vi "Teleop_Calc_Distance.vi"(11 "Teleop Local Data in":T1) -> (3 "Teleop Local Data out":T1)   [LabVIEW 2016]
uses:
  Typedefs/typedef_cluster_Teleop Local Data.ctl
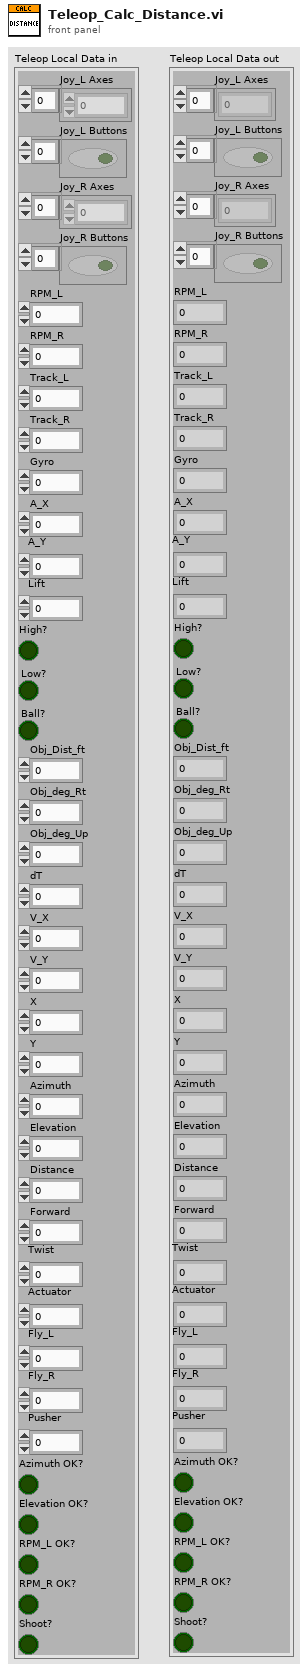
[diagram p1: front panel]
types:
  T1 = typedef "typedef_cluster_Teleop Local Data.ctl" = cluster{"Joy_L Axes":dbl[], "Joy_L Buttons":bool[], "Joy_R Axes":dbl[], "Joy_R Buttons":bool[], "RPM_L":dbl, "RPM_R":dbl, "Track_L":dbl, "Track_R":dbl, "Gyro":dbl, "A_X":dbl, "A_Y":dbl, "Lift":dbl, "High?":bool, "Low?":bool, "Ball?":bool, "Obj_Dist_ft":dbl, "Obj_deg_Rt":dbl, "Obj_deg_Up":dbl, "dT":dbl, "V_X":dbl, "V_Y":dbl, "X":dbl, "Y":dbl, "Azimuth":dbl, "Elevation":dbl, "Distance":dbl, "Forward":dbl, "Twist":dbl, "Actuator":dbl, "Fly_L":dbl, "Fly_R":dbl, "Pusher":dbl, "Azimuth OK?":bool, "Elevation OK?":bool, "RPM_L OK?":bool, "RPM_R OK?":bool, "Shoot?":bool}
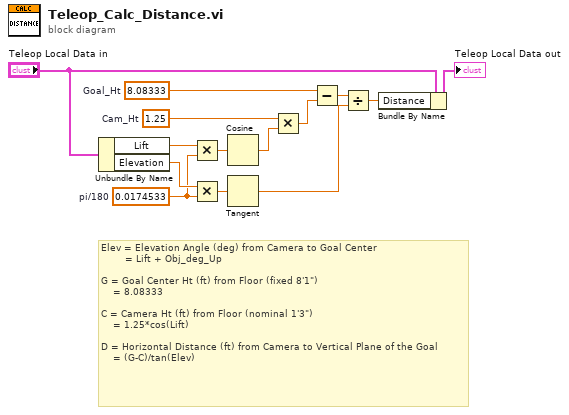
[diagram p0: block diagram]
diagram:
  w2 = 0.0174533  # pi/180
  w9 = 8.08333  # Goal_Ht
  w10 = 1.25  # Cam_Ht
  # "Elev = Elevation Angle (deg) from Camera to Goal Center\n        = Lift + Obj_deg_Up\n\nG = Goal Center Ht (ft) from Floor (fixed 8'1\")\n    = 8.08333\n\nC = Camera Ht (ft) from Floor (nominal 1'3\")\n    = 1.25*cos(Lift)\n\nD = Horizontal Distance (ft) from Camera to Vertical Plane of the Goal\n    = (G-C)/tan(Elev)"
  n1 = Unbundle By Name("Teleop Local Data in") -> ("Lift"=w12:dbl, "Elevation"=w7:dbl)
  n2 = Multiply(x=w12, y=w2) -> (x*y=w4:dbl)
  n3 = Multiply(x=w7, y=w2) -> (x*y=w3:dbl)
  n4 = Cosine(x=w4) -> (cos(x)=w11:dbl)
  n5 = Tangent(1:w3) -> (0:w5:dbl)
  n6 = Multiply(x=w10, y=w11) -> (x*y=w8:dbl)
  n7 = Subtract(x=w9, y=w8) -> (x-y=w6:dbl)
  n8 = Divide(x=w6, y=w5) -> (x/y=w1:dbl)
  n9 = Bundle By Name(cluster="Teleop Local Data in", "Distance"=w1) -> (→"Teleop Local Data out":T1)
